vi "Servo MSMT Set RF Power.vi"(8 "error in (no error)":errorcluster, 10 "Step In":refnum<k7>, 11 "Servo to Power Out in":refnum<class "Servo to Power Out.lvclass">) -> (0 "error out":errorcluster, 2 "Step Out":refnum<k7>, 3 "Servo to Power Out out":refnum<class "Servo to Power Out.lvclass">)   [LabVIEW 2018, in "Servo to Power Out.lvlib" / "Servo to Power Out.lvclass"]
uses:
  Servo to Power Out.lvclass
  C:/Sequence Automation/Plugins/Measurement Interface.lvlibp/Measurement Interface.lvclass
  C:/Sequence Automation/Plugins/Measurements/Servo MSMT.lvlibp/Measurements/Servo/Servo MSMT.lvclass
  Plugins/Measurement Interface.lvlibp/Private Methods/Measurement Parameters/Read Measurement Parameters.vi
  Plugins/String Database.lvlibp/String Database.lvclass
  Plugins/Measurements/Servo MSMT.lvlibp/Measurements/Servo/Servo MSMT.lvclass
  Plugins/Measurement Interface.lvlibp/Measurement Interface.lvclass
  Plugins/TestStand API Tools (TSAT).lvlibp/Step Actions/TSAT Step Actions.lvlib
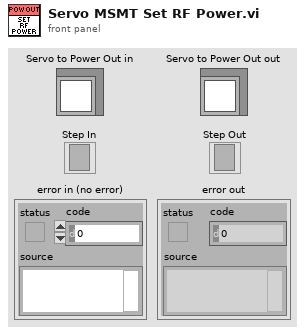
[diagram p1: front panel]
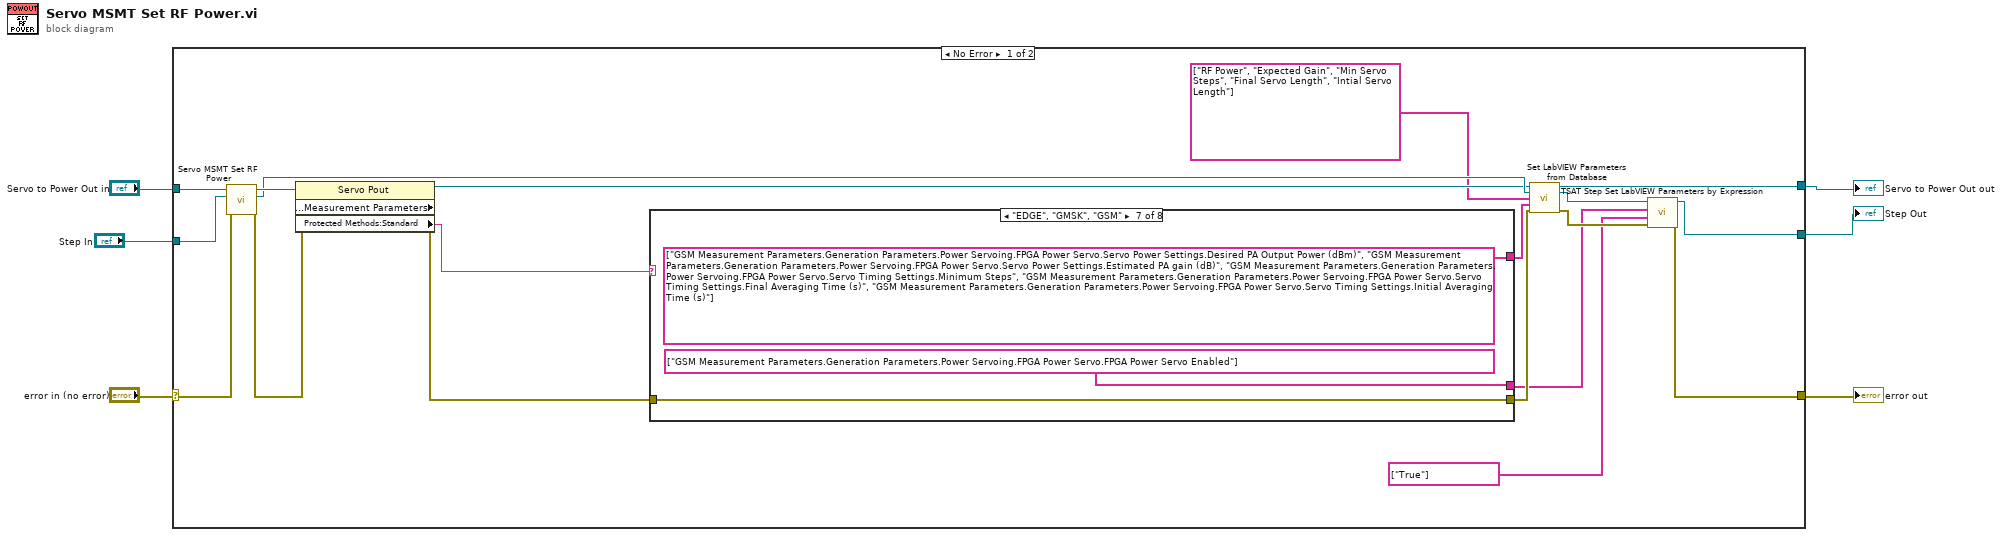
[diagram p0: block diagram]
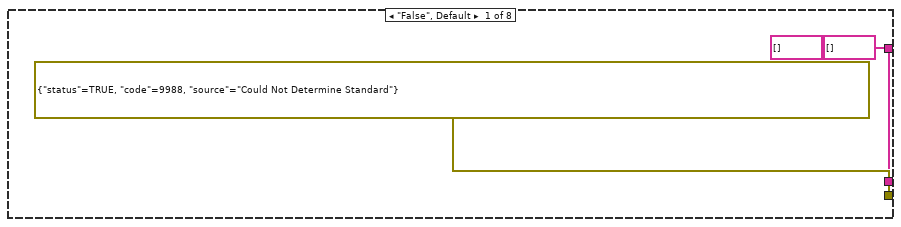
[diagram p2: hidden frame]
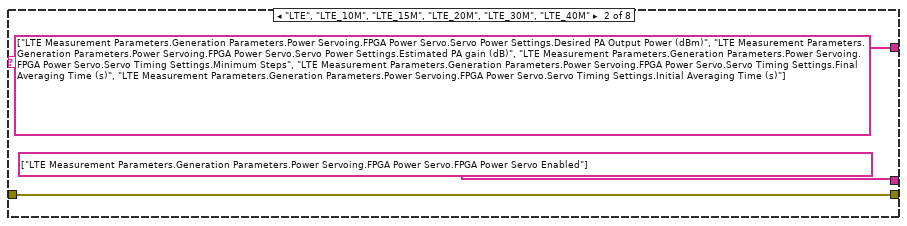
[diagram p3: hidden frame]
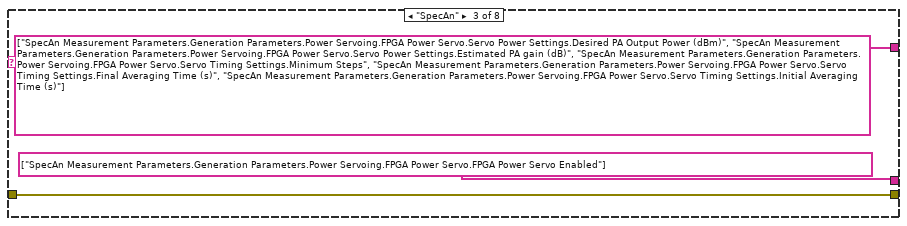
[diagram p4: hidden frame]
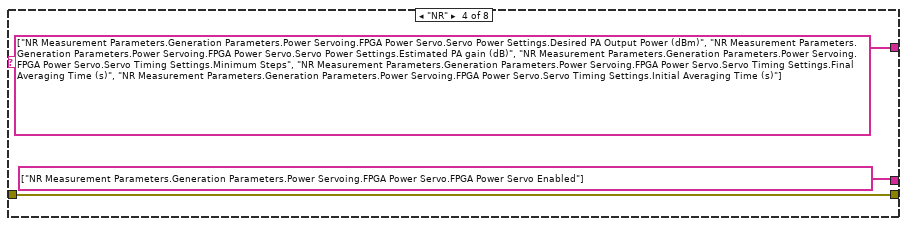
[diagram p5: hidden frame]
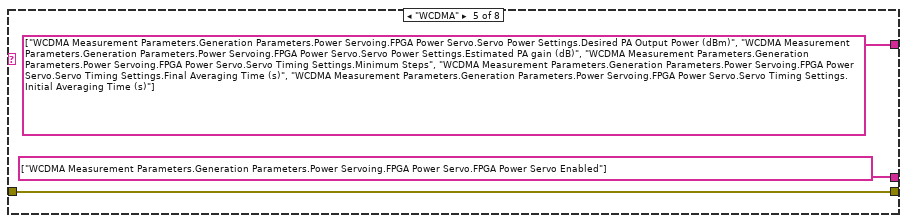
[diagram p6: hidden frame]
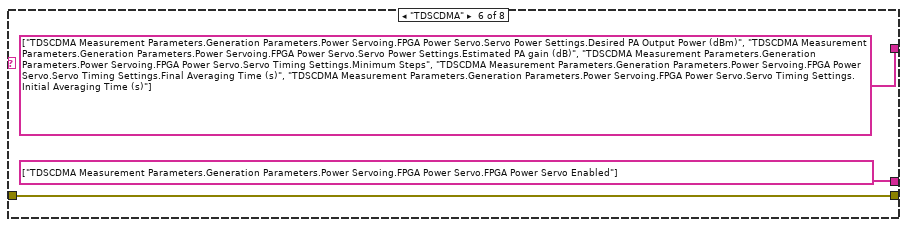
[diagram p7: hidden frame]
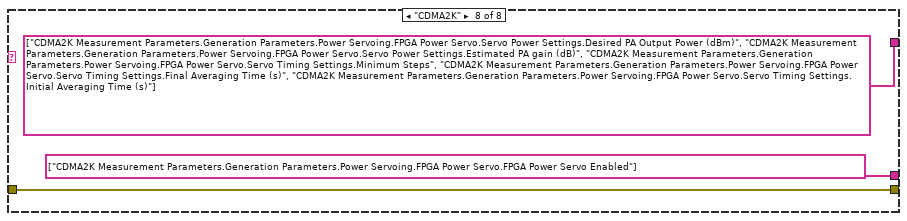
[diagram p8: hidden frame]
diagram:
  n1 = case shown="No Error" "error in (no error)" {
    selector: "error in (no error)" -> [w23 w50]
    tunnel: "Servo to Power Out in" -> [w21 w52]
    tunnel: [w15 w52] -> w5
    tunnel: "Step In" -> [w19 w51]
    tunnel: [w9 w50] -> w2
    tunnel: [w11 w51] -> w1
    frame No Error {
      n2 = call-parent "Servo MSMT Set RF Power.vi"("error in (no error)"=w23, "Step In"=w19, "Servo MSMT in"=w21) -> ("error out"=w22:errorcluster, "Step Out"=w18:refnum<k7>, "Servo MSMT out"=w20:refnum<class "Servo to Power Out.lvclass">)  [unwired: 6 in]
      n3 = property class="Servo Pout" props=["Protected Methods:Measurement Parameters", "Protected Methods:Standard"](reference=w20, error in=w22) -> (reference out=w16:refnum<class "Servo to Power Out.lvclass">, error out=w25:errorcluster, "Protected Methods:Standard"=w17:string)  [unwired: 1 out]
      n4 = case shown="\"EDGE\", \"GMSK\", \"GSM\"" w17 {
        tunnel: [errorcluster {"status"=TRUE, "code"=9988, "source"="Could Not Determine Standard"} ("error out") w31 w34 w37 w40 w43 w46 w49] -> w24
        tunnel: w25 -> [_ w31 w34 w37 w40 w43 w46 w49]
        tunnel: [string[] [] string[] ["LTE Measurement Parameters.Generation Parameters.Power Servoing.FPGA Power Servo.Servo Power Settings.Desired PA Output Power (dBm)", "LTE Measurement Parameters.Generation Parameters.Power Servoing.FPGA Power Servo.Servo Power Settings.Estimated PA gain (dB)", "LTE Measurement Parameters.Generation Parameters.Power Servoing.FPGA Power Servo.Servo Timing Settings.Minimum Steps", "LTE Measurement Parameters.Generation Parameters.Power Servoing.FPGA Power Servo.Servo Timing Settings.Final Averaging Time (s)", "LTE Measurement Parameters.Generation Parameters.Power Servoing.FPGA Power Servo.Servo Timing Settings.Initial Averaging Time (s)"] string[] ["SpecAn Measurement Parameters.Generation Parameters.Power Servoing.FPGA Power Servo.Servo Power Settings.Desired PA Output Power (dBm)", "SpecAn Measurement Parameters.Generation Parameters.Power Servoing.FPGA Power Servo.Servo Power Settings.Estimated PA gain (dB)", "SpecAn Measurement Parameters.Generation Parameters.Power Servoing.FPGA Power Servo.Servo Timing Settings.Minimum Steps", "SpecAn Measurement Parameters.Generation Parameters.Power Servoing.FPGA Power Servo.Servo Timing Settings.Final Averaging Time (s)", "SpecAn Measurement Parameters.Generation Parameters.Power Servoing.FPGA Power Servo.Servo Timing Settings.Initial Averaging Time (s)"] string[] ["NR Measurement Parameters.Generation Parameters.Power Servoing.FPGA Power Servo.Servo Power Settings.Desired PA Output Power (dBm)", "NR Measurement Parameters.Generation Parameters.Power Servoing.FPGA Power Servo.Servo Power Settings.Estimated PA gain (dB)", "NR Measurement Parameters.Generation Parameters.Power Servoing.FPGA Power Servo.Servo Timing Settings.Minimum Steps", "NR Measurement Parameters.Generation Parameters.Power Servoing.FPGA Power Servo.Servo Timing Settings.Final Averaging Time (s)", "NR Measurement Parameters.Generation Parameters.Power Servoing.FPGA Power Servo.Servo Timing Settings.Initial Averaging Time (s)"] string[] ["WCDMA Measurement Parameters.Generation Parameters.Power Servoing.FPGA Power Servo.Servo Power Settings.Desired PA Output Power (dBm)", "WCDMA Measurement Parameters.Generation Parameters.Power Servoing.FPGA Power Servo.Servo Power Settings.Estimated PA gain (dB)", "WCDMA Measurement Parameters.Generation Parameters.Power Servoing.FPGA Power Servo.Servo Timing Settings.Minimum Steps", "WCDMA Measurement Parameters.Generation Parameters.Power Servoing.FPGA Power Servo.Servo Timing Settings.Final Averaging Time (s)", "WCDMA Measurement Parameters.Generation Parameters.Power Servoing.FPGA Power Servo.Servo Timing Settings.Initial Averaging Time (s)"] string[] ["TDSCDMA Measurement Parameters.Generation Parameters.Power Servoing.FPGA Power Servo.Servo Power Settings.Desired PA Output Power (dBm)", "TDSCDMA Measurement Parameters.Generation Parameters.Power Servoing.FPGA Power Servo.Servo Power Settings.Estimated PA gain (dB)", "TDSCDMA Measurement Parameters.Generation Parameters.Power Servoing.FPGA Power Servo.Servo Timing Settings.Minimum Steps", "TDSCDMA Measurement Parameters.Generation Parameters.Power Servoing.FPGA Power Servo.Servo Timing Settings.Final Averaging Time (s)", "TDSCDMA Measurement Parameters.Generation Parameters.Power Servoing.FPGA Power Servo.Servo Timing Settings.Initial Averaging Time (s)"] string[] ["GSM Measurement Parameters.Generation Parameters.Power Servoing.FPGA Power Servo.Servo Power Settings.Desired PA Output Power (dBm)", "GSM Measurement Parameters.Generation Parameters.Power Servoing.FPGA Power Servo.Servo Power Settings.Estimated PA gain (dB)", "GSM Measurement Parameters.Generation Parameters.Power Servoing.FPGA Power Servo.Servo Timing Settings.Minimum Steps", "GSM Measurement Parameters.Generation Parameters.Power Servoing.FPGA Power Servo.Servo Timing Settings.Final Averaging Time (s)", "GSM Measurement Parameters.Generation Parameters.Power Servoing.FPGA Power Servo.Servo Timing Settings.Initial Averaging Time (s)"] string[] ["CDMA2K Measurement Parameters.Generation Parameters.Power Servoing.FPGA Power Servo.Servo Power Settings.Desired PA Output Power (dBm)", "CDMA2K Measurement Parameters.Generation Parameters.Power Servoing.FPGA Power Servo.Servo Power Settings.Estimated PA gain (dB)", "CDMA2K Measurement Parameters.Generation Parameters.Power Servoing.FPGA Power Servo.Servo Timing Settings.Minimum Steps", "CDMA2K Measurement Parameters.Generation Parameters.Power Servoing.FPGA Power Servo.Servo Timing Settings.Final Averaging Time (s)", "CDMA2K Measurement Parameters.Generation Parameters.Power Servoing.FPGA Power Servo.Servo Timing Settings.Initial Averaging Time (s)"]] -> w13
        tunnel: [string[] [] ("Parameters to Set") string[] ["LTE Measurement Parameters.Generation Parameters.Power Servoing.FPGA Power Servo.FPGA Power Servo Enabled"] ("Parameters to Set") string[] ["SpecAn Measurement Parameters.Generation Parameters.Power Servoing.FPGA Power Servo.FPGA Power Servo Enabled"] ("Parameters to Set") string[] ["NR Measurement Parameters.Generation Parameters.Power Servoing.FPGA Power Servo.FPGA Power Servo Enabled"] ("Parameters to Set") string[] ["WCDMA Measurement Parameters.Generation Parameters.Power Servoing.FPGA Power Servo.FPGA Power Servo Enabled"] ("Parameters to Set") string[] ["TDSCDMA Measurement Parameters.Generation Parameters.Power Servoing.FPGA Power Servo.FPGA Power Servo Enabled"] ("Parameters to Set") string[] ["GSM Measurement Parameters.Generation Parameters.Power Servoing.FPGA Power Servo.FPGA Power Servo Enabled"] ("Parameters to Set") string[] ["CDMA2K Measurement Parameters.Generation Parameters.Power Servoing.FPGA Power Servo.FPGA Power Servo Enabled"] ("Parameters to Set")] -> w8
        frame "False", Default {
        }
        frame "LTE", "LTE_10M", "LTE_15M", "LTE_20M", "LTE_30M", "LTE_40M" {
        }
        frame "SpecAn" {
        }
        frame "NR" {
        }
        frame "WCDMA" {
        }
        frame "TDSCDMA" {
        }
        frame "EDGE", "GMSK", "GSM" {
        }
        frame "CDMA2K" {
        }
      }
      n5 = call "Set LabVIEW Parameters from Database.vi"("Measurement Interface in"=w16, "Step In"=w18, "Dictionary Keys"=string[] ["RF Power", "Expected Gain", "Min Servo Steps", "Final Servo Length", "Intial Servo Length"], "LabVIEW Parameter Mapping"=w13, "error in (no error)"=w24) -> ("Measurement Interface out"=w15:refnum<class "Servo to Power Out.lvclass">, "Step Out"=w12:refnum<k7>, "error out"=w10:errorcluster)  [unwired: 8 in]
      n6 = call "TSAT Step Set LabVIEW Parameters by Expression.vi"("Error In"=w10, "Value Expressions"=string[] ["True"], "Parameters to Set"=w8, "Step In"=w12) -> ("Error Out"=w9:errorcluster, "Step Out"=w11:refnum<k7>)  [unwired: 6 in]
    }
    frame Error {
    }
  }
  "error out" <- w2
  "Servo to Power Out out" <- w5
  "Step Out" <- w1
